vi "numeric_indicator.vi"() -> ()   [LabVIEW 2020]
panel:
  out "Numeric 2":dbl
  out "k1":i32
  out "k2":i32
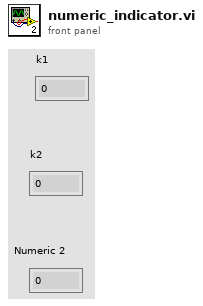
[diagram p1: front panel]
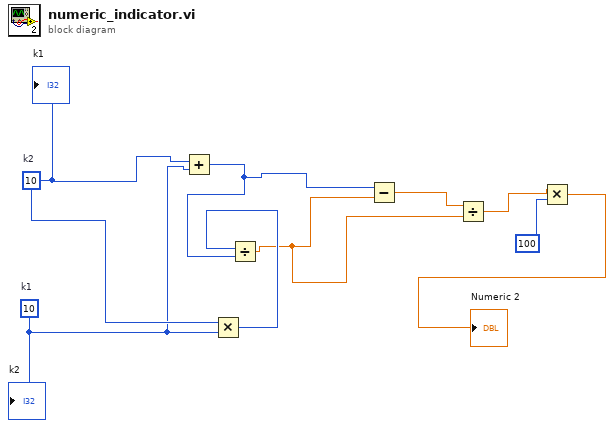
[diagram p0: block diagram]
diagram:
  w8 = 10  # k1
  w9 = 10  # k2
  n1 = Add(x=w9, y=w8) -> (x+y=w2:i32)
  n2 = Multiply(x=w9, y=w8) -> (x*y=w7:i32)
  n3 = Divide(x=w7, y=w2) -> (x/y=w1:dbl)
  n4 = Subtract(x=w2, y=w1) -> (x-y=w6:dbl)
  n5 = Divide(x=w6, y=w1) -> (x/y=w5:dbl)
  n6 = Multiply(x=w5, y=100) -> (x*y=→"Numeric 2":dbl)
  "k2" <- w8
  "k1" <- w9
